vi "ObjectTracking.vi"(7 "error in":errorcluster) -> (0 "error out":errorcluster, 1 "Frame Rate":dbl)   [LabVIEW 2016]
panel:
  out "Y Position":dbl(slide) scale=0.0..100.0
  out "X Position":dbl(slide) scale=0.0..100.0
  out "Ball Found":bool
  out "Nb Circles":i32
  out "Raw Circle Data":T1(array[cluster])
  out "Binary Image":T2(plugin-control)
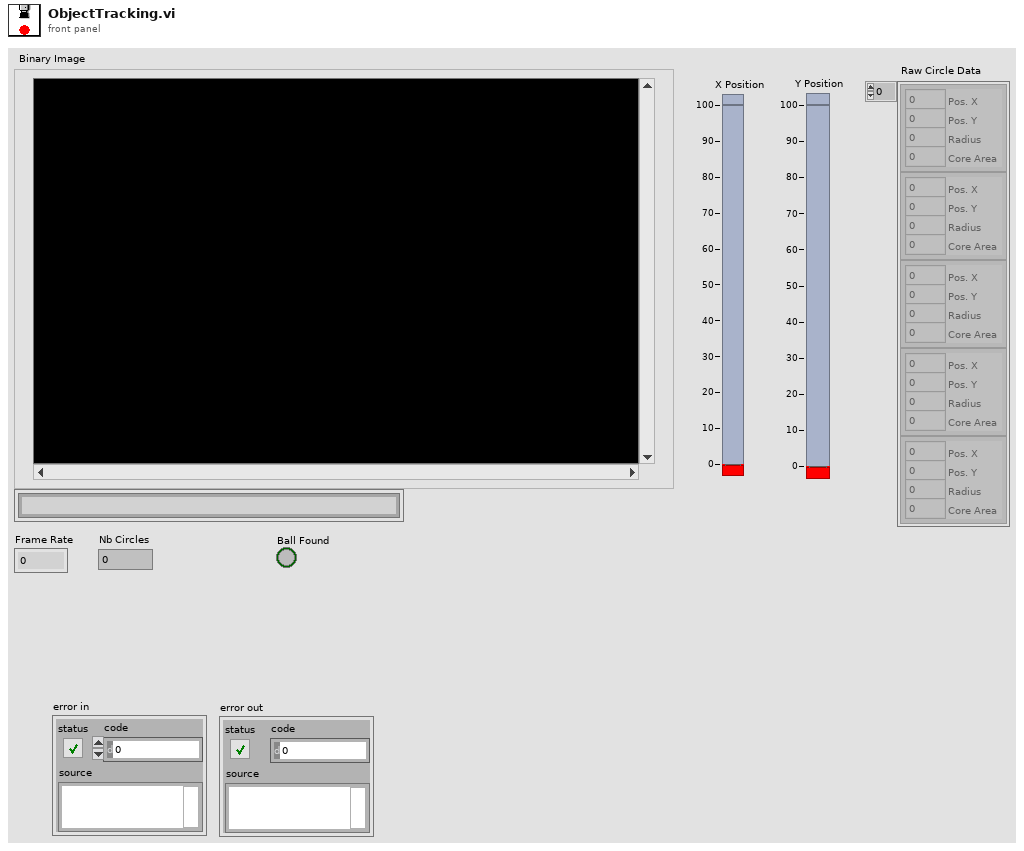
[diagram p1: front panel]
types:
  T1 = cluster{"Pos. X":i32, "Pos. Y":i32, "Radius":i32, "Core Area":i32}[]
  T2 = typedef "IMAQ Image.ctl" = refnum<image>
  T3 = cluster{"Pos. X":i32, "Pos. Y":i32, "Radius":i32, "Core Area":i32}
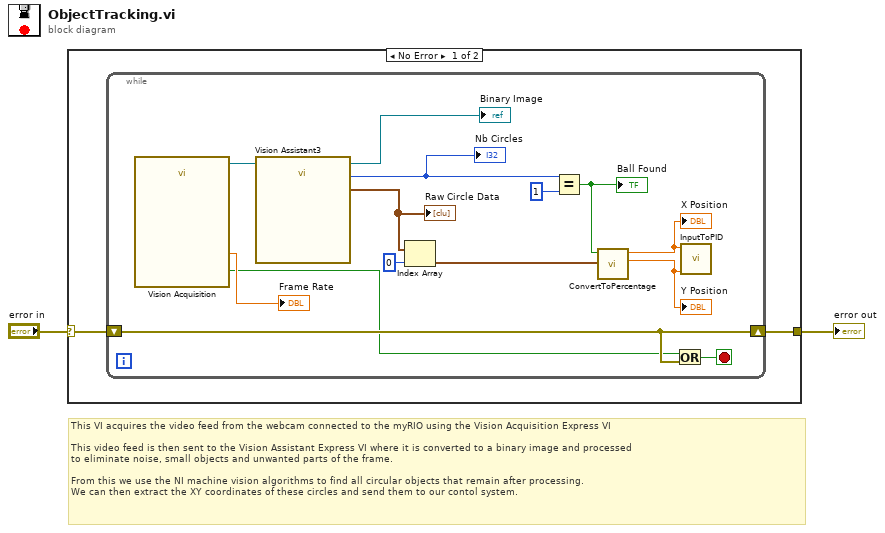
[diagram p0: block diagram]
diagram:
  # "This VI acquires the video feed from the webcam connected to the myRIO using the Vision Acquisition Express VI\n\nThis video feed is then sent to the Vision Assistant Express VI where it is converted to a binary image and processed\nto eliminate noise, small objects and unwanted parts of the frame.\n\nFrom this we use the NI machine vision algorithms to find all circular objects that remain after processing. \nWe can then extract the XY coordinates of these circles and send them to our contol system."
  n1 = case shown="No Error" "error in" {
    selector: "error in" -> [w3 w19]
    tunnel: [w4 w19] -> w2
    frame No Error {
      n2 = while {
        shift-right: [w17] -> w4
        shift-left: w3 -> [w17]
        stop <- w15 stop-if-true
        n3 = call "Vision Acquisition"() -> ("Image Out"=w14:T2, "Frame Rate"=→"Frame Rate":dbl, "Stopped"=w16:bool)  [unwired: 24 in, 1 out]
        n4 = call "Vision Assistant3"("Image In"=w14) -> ("Image Out"=→"Binary Image":T2, "Nb Circles (Circle Detection 1)"=w10:i32, "Circles Data (Circle Detection 1)"=w12:T1)  [unwired: 22 in, 2 out]
        "Raw Circle Data" <- w12
        "Nb Circles" <- w10
        n5 = Index Array(array=w12, index=0) -> (element=w7:T3)
        n6 = Equal?(x=w10, y=1) -> (x = y?=w8:bool)
        "Ball Found" <- w8
        n7 = call "ConvertToPercentage.vi"("Circles Data"=w7, "Boolean"=w8) -> ("Y Position"=w5:dbl, "X Position"=w6:dbl)  [unwired: 8 in]
        "X Position" <- w6
        "Y Position" <- w5
        n8 = Or(x=w16, y=w17) -> (x .or. y?=w15:bool)
        n9 = call "InputToPID.vi"("Y Position In"=w5, "X Position In"=w6) -> ()  [unwired: 8 in, 2 out]
      }
    }
    frame Error {
    }
  }
  "error out" <- w2
